vi "DAQmx(AI).METHOD_TEMPLATE.vi"(8 "error in (no error)":errorcluster, 10 "Data In":string, 11 "Subsystem":refnum<class "DAQmx(AI).lvclass">) -> (0 "error out":errorcluster, 2 "Data Out":string, 3 "Subsystem out":refnum<class "DAQmx(AI).lvclass">)   [LabVIEW 2013, in "DAQmx(AI).lvclass"]
doc: "---------------------------------------------------------------\nJKI State Machine Objects™\nhttp://jki.net/state-machine-objects/\nCopyright (C) 2005-2015, JKI <info@jki.net>\nALL RIGHTS RESERVEDJKI State Machine Objects (SMO) 1.0.0.5\nJKI - JKI\nCopyright (c) 2016, JKI"
uses:
  DAQmx(AI).lvclass
  DAQmx(AI).lvclass/DAQmx(AI).ctl
panel:
  # "For instructions on how to use the JKI State Machine Objects, examples and video tutorials, visit:\nhttp://jki.net/state-machine-objects/\n\nJKI State Machine Objects™\nhttp://jki.net/state-machine-objects/\nCopyright (C) 2005-2015, JKI <info@jki.net>\nALL RIGHTS RESERVED"
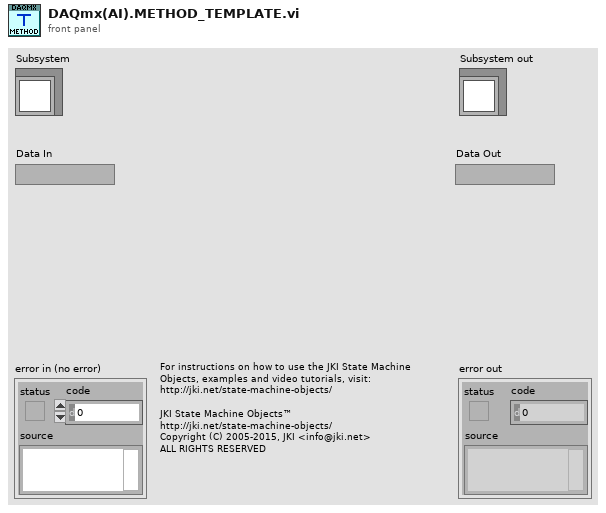
[diagram p1: front panel]
types:
  T1 = typedef "DAQmx(AI).lvclass/PrivateData--Ref.ctl" = refnum<data-value>
  T2 = typedef "DAQmx(AI).lvclass/PrivateData--Cluster.ctl" = cluster{"Configuration":T3, "Public Events":T5, "Data":dbl, "Scaling":T6}
  T3 = typedef "DAQmx(AI).lvclass/Configuration--Cluster.ctl" = cluster{"PhysChan":tag, "Period (ms)":i64, "input terminal cfg":i32, "minimum value":dbl, "maximum value":dbl, "units":T4, "task name":string}
  T4 = typedef "DAQmx(AI).lvclass/Units -- Enum.ctl" = enum16{"Volts", "Amps", "Deg F", "Deg C", "Deg R", "Kelvins", "Strain", "Ohms", "Hz", "Seconds", "Meters", "Inches", "Degrees", "Radians", "Ticks", "g", "m/s^2", "m/s", "in/s", "Pascals", "Newtons", "Pounds", "kgf", "psi", "bar", "Nm", "oz-in", "lb-in", "lb-ft", "Volts/Volt", "mVolts/Volt", "From TEDS"}
  T5 = typedef "DAQmx(AI).lvclass/PublicEvents--Cluster.ctl" = cluster{"Value Changed":refnum<user-event>, "Task Configuration":refnum<user-event>, "Scaling":refnum<user-event>}
  T6 = typedef "DAQmx(AI).lvclass/Scaling--Cluster.ctl" = cluster{"Scale Name":string, "Scale Type":T7, "Scaled Units":string, "Linear":T8, "Map Range":T9, "Polynomial":T10, "Table":T11}
  T7 = typedef "DAQmx(AI).lvclass/ScalingType--Enum.ctl" = enum16{"No scaling", "Linear", "Map Range", "Polynomial", "Table"}
  T8 = typedef "DAQmx(AI).lvclass/Scaling(Linear)--Cluster.ctl" = cluster{"Slope":dbl, "Intercept":dbl}
  T9 = typedef "DAQmx(AI).lvclass/Scaling(MapRange)--Cluster.ctl" = cluster{"Minimum":dbl, "Maximum":dbl}
  T10 = typedef "DAQmx(AI).lvclass/Scaling(Polynomial)--Cluster.ctl" = cluster{"forward coeff":dbl[], "reverse coeff":dbl[]}
  T11 = typedef "DAQmx(AI).lvclass/Scaling(Table)--Cluster.ctl" = cluster{"scaled values":dbl[], "pres-scaled values":dbl[]}
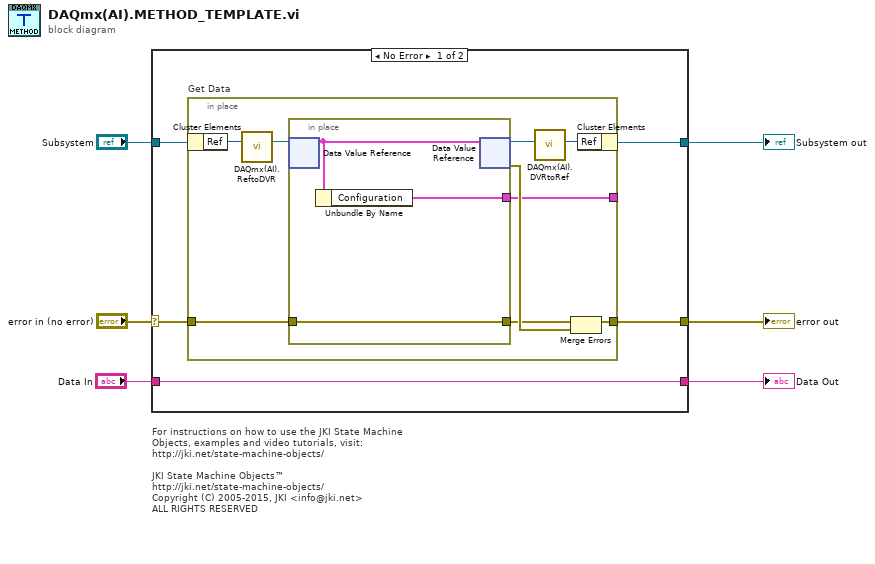
[diagram p0: block diagram]
diagram:
  # "For instructions on how to use the JKI State Machine Objects, examples and video tutorials, visit:\nhttp://jki.net/state-machine-objects/\n\nJKI State Machine Objects™\nhttp://jki.net/state-machine-objects/\nCopyright (C) 2005-2015, JKI <info@jki.net>\nALL RIGHTS RESERVED"
  n1 = case shown="No Error" "error in (no error)" {
    selector: "error in (no error)" -> [w10 w25]
    tunnel: "Subsystem" -> [w11 w26]
    tunnel: [w7 w25] -> w5
    tunnel: [w8 w26] -> w4
    tunnel: [w9 w24] -> w2
    tunnel: "Data In" -> [w9 w24]
    frame No Error {
      n2 = in-place "Get Data" {
        in-place-border: w10 -> [w20]
        in-place-border: [w17] -> w7
        in-place-border: [w12] -> _
        n3 = in-place-cluster #1(w11) -> ("Ref"=w16:u32)
        n4 = call "DAQmx(AI).ReftoDVR.vi"("Ref"=w16) -> ("Ref"=w15:T1)  [unwired: 10 in]
        n5 = in-place {
          in-place-border: w20 -> [w22]
          in-place-border: [w22] -> w18
          in-place-border: [w21] -> w12
          n6 = in-place-dvr #2(w15) -> (w23:T2)  [unwired: 1 out]
          n7 = Unbundle By Name(w23) -> ("Configuration"=w21:T3)
          n8 = in-place-dvr #2(w23) -> (w14:T1, w19:errorcluster)
        }
        n9 = call "DAQmx(AI).DVRtoRef.vi"("Ref"=w14) -> ("Ref"=w13:u32)  [unwired: 10 in]
        n10 = Merge Errors(w18, w19) -> (w17:errorcluster)
        n11 = in-place-cluster #1("Ref"=w13) -> (w8:refnum<class "DAQmx(AI).lvclass">)
      }
    }
    frame Error {
    }
  }
  "error out" <- w5
  "Subsystem out" <- w4
  "Data Out" <- w2
